vi "FPPVv2.vi"(0 "instrument handle":refnum<k15>="PXI1Slot2 (59)", 1 "Max attempts":dbl=2000.0 format="%#_13g", 2 "MLC BLV (V)":dbl=2.0, 5 "Lower resistance (ohm)":dbl, 9 "Upper resistance (ohm)":dbl=6000.0, 11 "error in (no error)":errorcluster, 13 "MLC WLV (V)":dbl=3.0) -> (3 "SL voltage (V)":dbl, 4 "instrument handle out":refnum<k15>="PXI1Slot2 (59)", 6 "final resistance (ohm)":dbl=1580290.44017172 format="%#_6p", 8 "target hit?":bool=TRUE, 10 "final current (A)":dbl=1.265590140368547e-07, 12 "BL voltage (V)":dbl=2.0, 14 "WL voltage (V)":dbl=3.0, 15 "error out":errorcluster)   [LabVIEW 2018]
panel:
  out "attempt number":i32
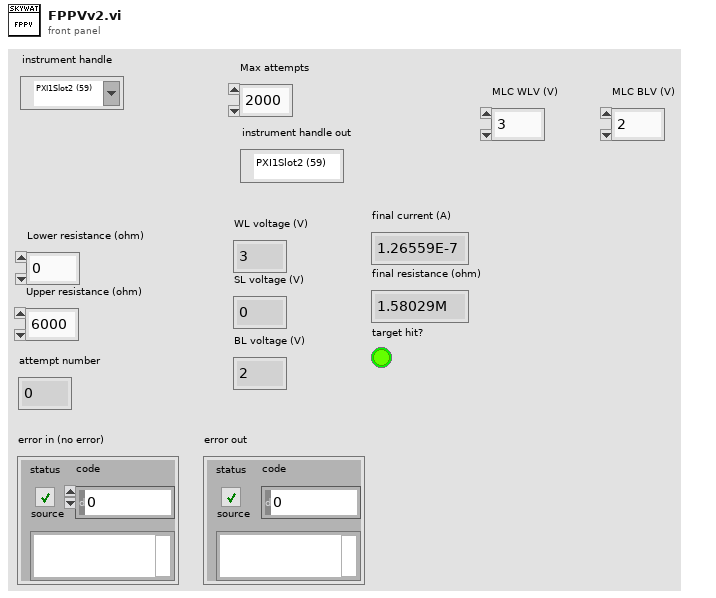
[diagram p1: front panel]
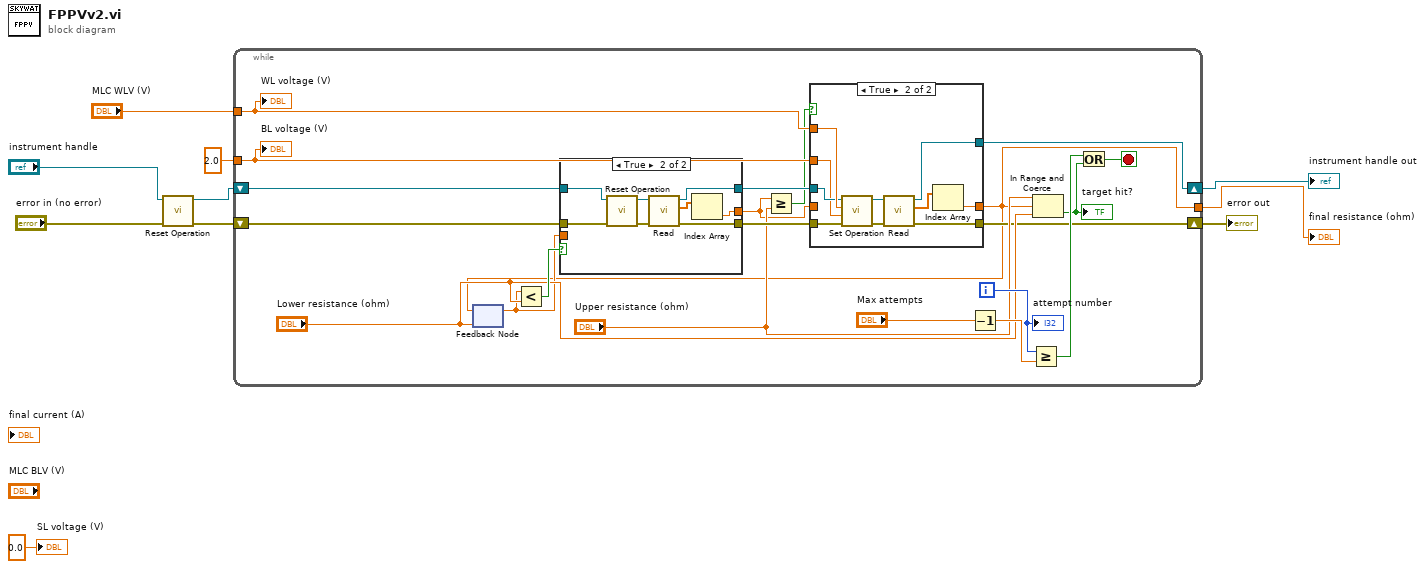
[diagram p0: block diagram]
diagram:
  n1 = call "Reset Operation.vi"("error in (no error)"="error in (no error)", "instrument handle"="instrument handle") -> ("error out"=w5:errorcluster, "instrument handle out"=w4:refnum<k15>)  [unwired: 8 in]
  n2 = while {
    shift-right: [w13] -> w10
    shift-left: w4 -> [w20]
    shift-right: [w14] -> w9
    shift-left: w5 -> [w19]
    tunnel: "MLC WLV (V)" -> [w29]
    tunnel: [w11] -> w1
    tunnel: 2.0 ("MLC BLV (V)") -> [w24]
    i -> [w31]
    stop <- w28 stop-if-true
    n3 = feedback #1("Lower resistance (ohm)") -> (w17:dbl)
    n4 = Less?(x=w17, y="Lower resistance (ohm)") -> (x < y?=w21:bool)
    n5 = case shown="True" w21 {
      tunnel: [w46 w51] -> w27
      tunnel: [w47 w52] -> w26
      tunnel: w20 -> [w47 w55]
      tunnel: w19 -> [w46 w54]
      tunnel: w17 -> [w45 _]
      tunnel: [w45 w48] -> w12
      frame False {
      }
      frame True {
        n6 = call "Reset Operation.vi"("error in (no error)"=w54, "instrument handle"=w55) -> ("error out"=w50:errorcluster, "instrument handle out"=w53:refnum<k15>)  [unwired: 8 in]
        n7 = call "Read.vi"("error in (no error)"=w50, "instrument handle"=w53) -> ("error out"=w51:errorcluster, "resistances (ohm)"=w49:dbl[], "instrument handle out"=w52:refnum<k15>)  [unwired: 6 in, 1 out]
        n8 = Index Array(array=w49) -> (element=w48:dbl)  [unwired: 1 in]
      }
    }
    n9 = Greater Or Equal?(x=w12, y="Upper resistance (ohm)") -> (x >= y?=w15:bool)
    n10 = case shown="True" w15 {
      tunnel: w29 -> [_ w44]
      tunnel: w27 -> [w33 w43]
      tunnel: w26 -> [w34 w42]
      tunnel: w24 -> [_ w41]
      tunnel: [w33 w38] -> w14
      tunnel: [w34 w37] -> w13
      tunnel: [w32 w35] -> w11
      tunnel: w12 -> [w32 _]
      frame False {
      }
      frame True {
        n11 = call "Set Operation.vi"("error in (no error)"=w43, "BLV"=w41, "WLV"=w44, "instrument handle"=w42) -> ("error out"=w40:errorcluster, "instrument handle out"=w39:refnum<k15>)  [unwired: 6 in]
        n12 = call "Read.vi"("error in (no error)"=w40, "instrument handle"=w39) -> ("error out"=w38:errorcluster, "resistances (ohm)"=w36:dbl[], "instrument handle out"=w37:refnum<k15>)  [unwired: 6 in, 1 out]
        n13 = Index Array(array=w36) -> (element=w35:dbl)  [unwired: 1 in]
      }
    }
    n14 = feedback-in #1(w11) -> ()
    n15 = Decrement(x="Max attempts") -> (x-1=w22:dbl)
    n16 = Greater Or Equal?(x=w31, y=w22) -> (x >= y?=w30:bool)
    n17 = In Range and Coerce(upper limit="Upper resistance (ohm)", x=w11, lower limit="Lower resistance (ohm)") -> (In Range?=w25:bool)  [unwired: 1 out]
    "target hit?" <- w25
    n18 = Or(x=w30, y=w25) -> (x .or. y?=w28:bool)
    "attempt number" <- w31
    "WL voltage (V)" <- w29
    "BL voltage (V)" <- w24
  }
  "error out" <- w9
  "instrument handle out" <- w10
  "final resistance (ohm)" <- w1
  "SL voltage (V)" <- 0.0 ("SL voltage (V)")
